vi "crio_FPGA_LAC_PWM_control.vi"() -> ()   [LabVIEW 2019]
uses:
  <vilib>/rvi/Emulation/niFpgaSctlEmulationGetInTimedLoop.vi
  <vilib>/rvi/Emulation/niFpgaProcessEmulError.vi
  <vilib>/rvi/eio/common/nirviEmuTemplateMethod_errors.vi
  <vilib>/rvi/Emulation/niFpgaGetClockAttributes.vi
  <vilib>/rvi/Emulation/niFpgaEmulationReportErrorSimple.vi
  <vilib>/rvi/Emulation/niFpgaCriticalErrorInLSC.vi
  <vilib>/eio/EIOMethodNode/EIOMethodNode.xnode
  <vilib>/eio/EIONode/EIONode.xnode
panel:
  in  "LAC Lock":bool
  in  "Duty Cycle":sgl(slide) scale=0.0..1.0
  in  "Debug: ConnectorA/DIO15":bool
  in  "Debug: ConnectorA/DIO14":bool
  in  "Encoder Debug":bool
  in  "Loop Timer DAQ":u32=1 caption="Loop Time(uSec)"
  in  "Position Reset":bool
  out "Position (Counts)":i32
  out "B":bool
  out "A":bool
  out "B'":bool
  out "A'":bool
  in  "Velocity Interval (uSec)":u32=1000
  out "Acceleration (Counts/Interval)":i32
  out "Velocity (Counts/Interval)":i32
  in  "stop":bool
  in  "Period  (us)":u32=2000
  # "0, fully retract\n1, fully extend\nbetween, inner PD control"
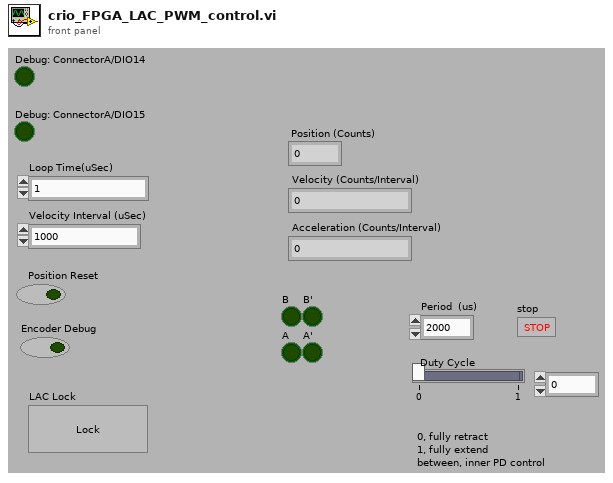
[diagram p1: front panel]
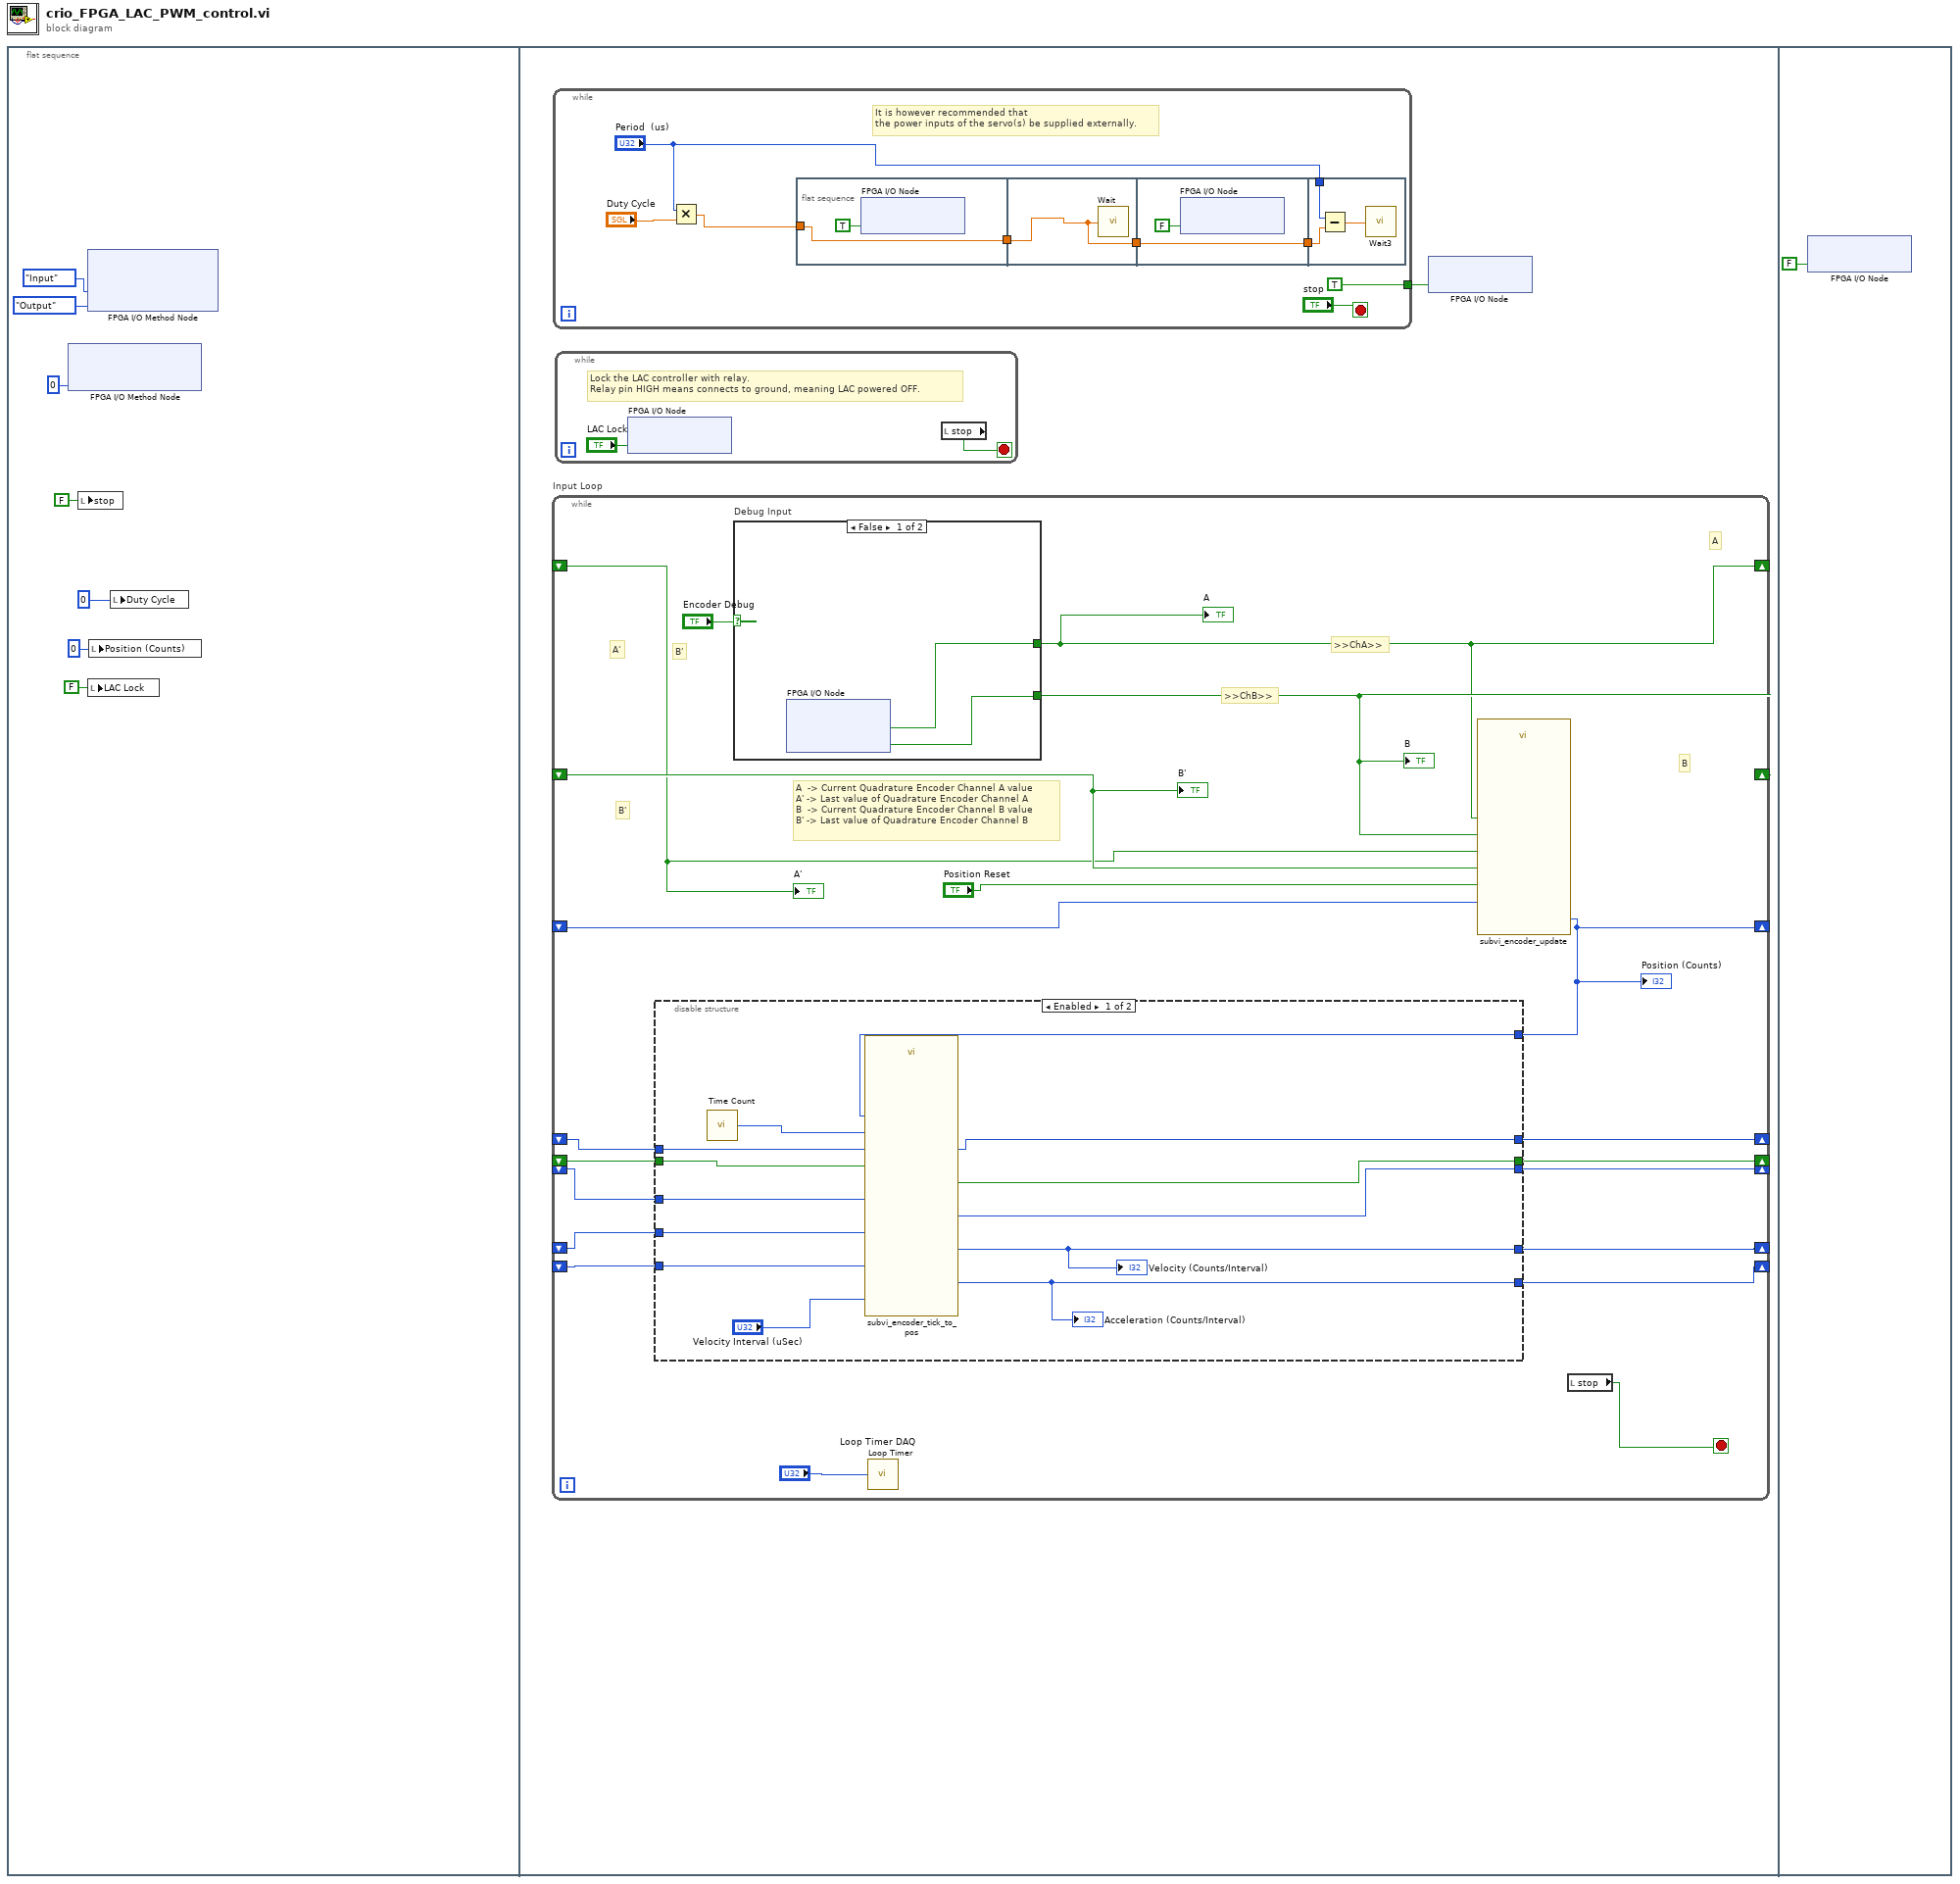
[diagram p0: block diagram]
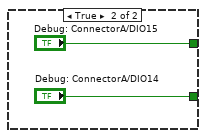
[diagram p3: hidden frame]
diagram:
  n1 = flat-sequence {
    frame #0 {
      n2 = xnode "FPGA I/O Method Node"("Enable"=u8 0) -> ()  [unwired: 1 in, 1 out]
      n3 = local write "stop"(FALSE ("stop")) -> ()
      n4 = xnode "FPGA I/O Method Node"("DIO 7:4"=enum8{"No Change", "Input", "Output"}."Input", "DIO 3:0"=enum8{"No Change", "Input", "Output"}."Output") -> ()  [unwired: 1 in, 1 out]
      n5 = local write "LAC Lock"(FALSE ("LAC Lock")) -> ()
      n6 = local write "Position (Counts)"(0 ("Position (Counts)")) -> ()
      n7 = local write "Duty Cycle"(u32 0 ("Servo wait time")) -> ()
    }
    frame #1 {
      n8 = while "Input Loop" {
        shift-right: [w24] -> _
        shift-left: _ -> [w27]
        shift-right: [w23] -> _
        shift-left: _ -> [w26]
        shift-right: [w19] -> _
        shift-left: _ -> [w25]
        shift-right: [w12] -> _
        shift-left: _ -> [w22]
        shift-right: [w13] -> _
        shift-left: _ -> [w21]
        shift-right: [w20] -> _
        shift-left: _ -> [w18]
        shift-right: [w17] -> _
        shift-left: _ -> [w16]
        shift-right: [w15] -> _
        shift-left: _ -> [w14]
        stop <- w11 stop-if-true
        # "B'"
        # ">>ChB>>"
        # ">>ChA>>"
        # "A'"
        # "A  -> Current Quadrature Encoder Channel A value\nA' -> Last value of Quadrature Encoder Channel A\nB  -> Current Quadrature Encoder Channel B value\nB' -> Last value of Quadrature Encoder Channel B"
        # "B'"
        # "B"
        # "A"
        n9 = case "Debug Input" shown="False" "Encoder Debug" {
          tunnel: [w45 "Debug: ConnectorA/DIO15"] -> w23
          tunnel: [w44 "Debug: ConnectorA/DIO14"] -> w24
          frame False {
            n10 = xnode "FPGA I/O Node"() -> ("Mod2/DIO2"=w45:bool, "Mod2/DIO3"=w44:bool)  [unwired: 2 in, 2 out]
          }
          frame True {
          }
        }
        "B" <- w24
        "A" <- w23
        n11 = call "Loop Timer"("Count(uSec)"="Loop Timer DAQ") -> ()  [unwired: 1 out]
        n12 = call "subvi_encoder_update.vi"("Position Reset"="Position Reset", "Tick'"=w25, "A"=w23, "B'"=w27, "A'"=w26, "B"=w24) -> ("Tick"=w19:i32)  [unwired: 5 in]
        "Position (Counts)" <- w19
        n13 = disable-structure shown="Enabled" {
          disable-tunnel: w22 -> [w42 _]
          disable-tunnel: w21 -> [w41 _]
          disable-tunnel: [w40 _] -> w20
          disable-tunnel: w19 -> [w39 _]
          disable-tunnel: w18 -> [w38 _]
          disable-tunnel: [w37 _] -> w17
          disable-tunnel: w16 -> [w36 _]
          disable-tunnel: [w35 _] -> w15
          disable-tunnel: w14 -> [w34 _]
          disable-tunnel: [w32 _] -> w13
          disable-tunnel: [w31 _] -> w12
          frame Enabled {
            n14 = call "Time Count"() -> ("Tick Count(uSec)"=w33:u32)
            n15 = call "subvi_encoder_tick_to_pos.vi"("Velocity Interval (uSec)"="Velocity Interval (uSec)", "Raw Tick"=w39, "Waited?'"=w36, "Tick Count(uSec)'"=w34, "p'"=w38, "Time Count"=w33, "a'"=w41, "v'"=w42) -> ("Waited?"=w37:bool, "Tick Count(uSec)"=w35:u32, "p"=w40:i32, "a"=w32:i32, "v"=w31:i32)  [unwired: 3 in]
            "Acceleration (Counts/Interval)" <- w32
            "Velocity (Counts/Interval)" <- w31
          }
          frame Disabled {
          }
        }
        n16 = local read "stop"() -> (w11:bool)
        "B'" <- w27
        "A'" <- w26
      }
      n17 = while {
        tunnel: [TRUE] -> w8
        stop <- "stop" stop-if-true
        # "It is however recommended that\nthe power inputs of the servo(s) be supplied externally."
        n18 = Multiply(x="Period  (us)", y="Duty Cycle") -> (x*y=w50:sgl)
        n19 = flat-sequence {
          tunnel: w50 -> [w56]
          tunnel: [w56] -> w49
          tunnel: [w58] -> w52
          tunnel: w49 -> [w58]
          tunnel: [w59] -> w53
          tunnel: w52 -> [w59]
          tunnel: "Period  (us)" -> [w63]
          tunnel: w53 -> [w62]
          frame #0 {
            n20 = xnode "FPGA I/O Node"("Mod8/DIO5"=TRUE) -> ()  [unwired: 1 in, 1 out]
          }
          frame #1 {
            n21 = call "Wait"("Count(uSec)"=w58) -> ()  [unwired: 1 out]
          }
          frame #2 {
            n22 = xnode "FPGA I/O Node"("Mod8/DIO5"=FALSE) -> ()  [unwired: 1 in, 1 out]
          }
          frame #3 {
            n23 = Subtract(x=w63, y=w62) -> (x-y=w61:sgl)
            n24 = call "Wait3"("Count(uSec)"=w61) -> ()  [unwired: 1 out]
          }
        }
      }
      n25 = while {
        stop <- w10 stop-if-true
        # "Lock the LAC controller with relay.\nRelay pin HIGH means connects to ground, meaning LAC powered OFF."
        n26 = xnode "FPGA I/O Node"("Mod8/DIO6"="LAC Lock") -> ()  [unwired: 1 in, 1 out]
        n27 = local read "stop"() -> (w10:bool)
      }
      n28 = xnode "FPGA I/O Node"("Mod8/DIO5"=w8) -> ()  [unwired: 1 in, 1 out]
    }
    frame #2 {
      n29 = xnode "FPGA I/O Node"("Mod8/DIO5"=FALSE) -> ()  [unwired: 1 in, 1 out]
    }
  }
